vi "Event-Timestep.vi"(7 "Timestep":i32, 8 "error in (no error)":errorcluster, 10 "Data ref. in":refnum<data-value>, 11 "UI ref. in":refnum<data-value>) -> (0 "error out":errorcluster, 2 "Data ref.":refnum<data-value>, 3 "UI ref.":refnum<data-value>)   [LabVIEW 2013, in "CameraVision.lvlib" / "CV-UI.lvclass"]
uses:
  CV-UI.lvclass
  Main/CV-Main.lvclass
  CV-UI.lvclass/CV-UI.ctl
  Main/Main-actions.ctl
  Read Timestep.vi
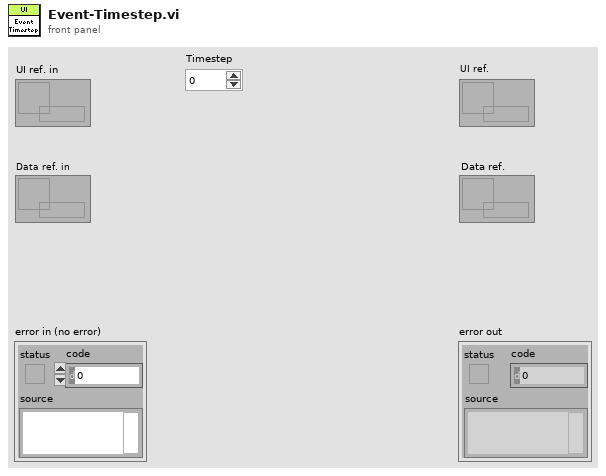
[diagram p1: front panel]
types:
  T1 = typedef "CameraVision.lvlib/CV-Main.lvclass/Main-actions.ctl" = enum16{"Idle", "Initialize", "Load defaults", "Update settings", "Check settings", "Save settings", "Save settings with dialog", "Load settings", "Load data", "Activate", "Start", "Wait for start signal", "Acquire & process", "Iterate", "Stop", "Refresh display", "Refresh status", "View camera settings", "View grabber settings", "Exit"}
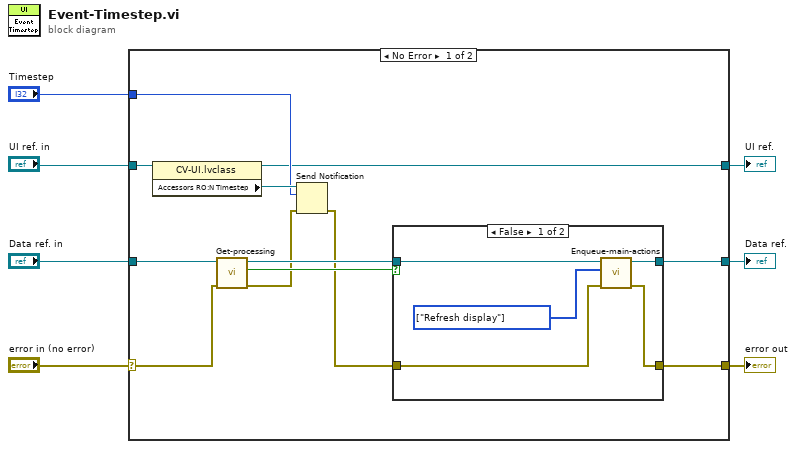
[diagram p0: block diagram]
diagram:
  n1 = case shown="No Error" "error in (no error)" {
    selector: "error in (no error)" -> [w14 w29]
    tunnel: [w17 w29] -> w6
    tunnel: [w8 w28] -> w4
    tunnel: "UI ref. in" -> [w13 w28]
    tunnel: "Data ref. in" -> [w19 w27]
    tunnel: "Timestep" -> [w9 _]
    tunnel: [w15 w27] -> w1
    frame No Error {
      n2 = property class="CV-UI.lvclass"(reference=w13) -> (reference out=w8:refnum<data-value>, "Accessors RO:N Timestep"=w12:refnum<notifier>)  [unwired: 1 in, 1 out]
      n3 = call "Get-processing.vi"("error in (no error)"=w14, "Data ref. in"=w19) -> ("error out"=w11:errorcluster, "Processing?"=w18:bool, "Data ref."=w16:refnum<data-value>)  [unwired: 7 in]
      n4 = Send Notification(notification=w9, notifier=w12, error in (no error)=w11) -> (error out=w10:errorcluster)  [unwired: 1 out]
      n5 = case shown="False" w18 {
        tunnel: w10 -> [w22 w26]
        tunnel: [w23 w26] -> w17
        tunnel: w16 -> [w21 w25]
        tunnel: [w20 w25] -> w15
        frame False {
          w24 = T1[] [enum."Refresh display"] items=["Idle", "Initialize", "Load defaults", "Update settings", "Check settings", "Save settings", "Save settings with dialog", "Load settings", "Load data", "Activate", "Start", "Wait for start signal", "Acquire & process", "Iterate", "Stop", "Refresh display", "Refresh status", "View camera settings", "View grabber settings", "Exit"] ("State array")
          n6 = call "Enqueue-main-actions.vi"("error in (no error)"=w22, "State array"=w24, "Data ref. in"=w21) -> ("error out"=w23:errorcluster, "Data ref."=w20:refnum<data-value>)  [unwired: 6 in, 1 out]
        }
        frame True {
        }
      }
    }
    frame Error {
    }
  }
  "error out" <- w6
  "Data ref." <- w1
  "UI ref." <- w4
